vi "HEWH Check Quick Skip.vi"(8 "Error In":errorcluster, 9 "Condition#":T1, 10 "Current Cond":T1, 11 "Saved Condition Read":T1) -> (0 "Error Out":errorcluster, 3 "Quick Skip?":bool)   [LabVIEW 2019]
uses:
  Draw Water Specific/Type Definitions/HEWH Special Condition Check.ctl
panel:
  out "x = y? 2":bool
  out "x = y?":bool
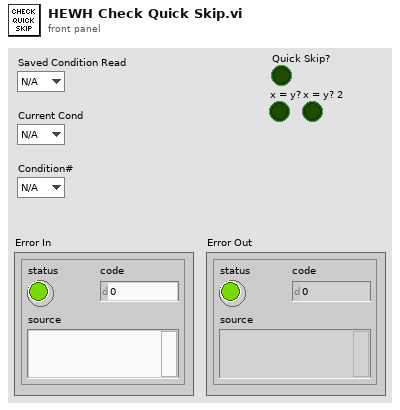
[diagram p1: front panel]
types:
  T1 = typedef "HEWH Special Condition Check.ctl" = enum16{"N/A", "C1", "C2", "Reset/Fail", "Skip Draw Sequence"}
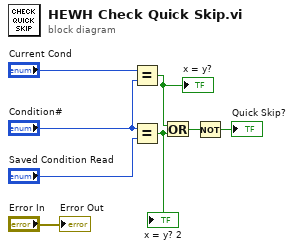
[diagram p0: block diagram]
diagram:
  n1 = Equal?(x="Current Cond", y="Condition#") -> (x = y?=w6:bool)
  "x = y?" <- w6
  n2 = Equal?(x="Condition#", y="Saved Condition Read") -> (x = y?=w7:bool)
  "x = y? 2" <- w7
  n3 = Or(x=w6, y=w7) -> (x .or. y?=w8:bool)
  n4 = Not(x=w8) -> (.not. x?=→"Quick Skip?":bool)
  "Error Out" <- "Error In"
